vi "Tool_Unicode Update Caption.vi"(5 "Interpret as Unicode (T)":bool=TRUE, 6 "error in (no error)":errorcluster, 7 "Caption":string, 9 "Control Reference":refnum<vi>) -> (0 "error out":errorcluster, 3 "Control Reference":refnum<vi>)   [LabVIEW 2020]
doc: "Apply a caption text to the specified control/indicator. Interpret string as Unicode is set."
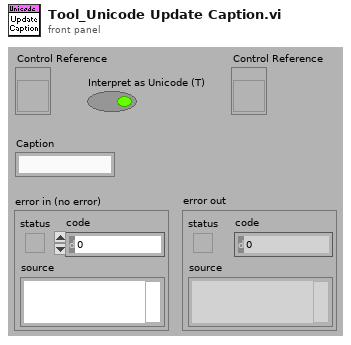
[diagram p1: front panel]
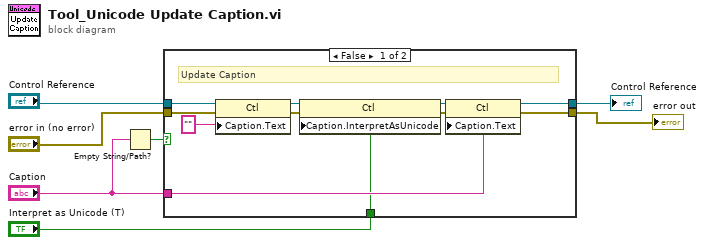
[diagram p0: block diagram]
diagram:
  n1 = Empty String/Path?(string/path="Caption") -> (empty?=w6:bool)
  n2 = case shown="False" w6 {
    tunnel: "Control Reference" -> [w16 w20]
    tunnel: "error in (no error)" -> [w13 w19]
    tunnel: "Caption" -> [w12 _]
    tunnel: [w18 w20] -> w1
    tunnel: [w17 w19] -> w2
    tunnel: "Interpret as Unicode (T)" -> [w10 _]
    frame False {
      # "Update Caption"
      n3 = property class="Ctl"(reference=w16, error in=w13, "Caption.Text"="") -> (reference out=w15:refnum<vi>, error out=w14:errorcluster)
      n4 = property class="Ctl"(reference=w15, error in=w14, "Caption.InterpretAsUnicode"=w10) -> (reference out=w9:refnum<vi>, error out=w8:errorcluster)
      n5 = property class="Ctl"(reference=w9, error in=w8, "Caption.Text"=w12) -> (reference out=w18:refnum<vi>, error out=w17:errorcluster)
    }
    frame True {
    }
  }
  "error out" <- w2
  "Control Reference" <- w1
